vi "laserChangePara.vi"(7 "LaserProp":T1, 8 "error in (no error)":errorcluster, 9 "LaserMode":string, 10 "LaserON":bool, 11 "LaserPow":dbl) -> (0 "error out":errorcluster, 2 "String":string, 3 "Boolean":bool)   [LabVIEW 2021]
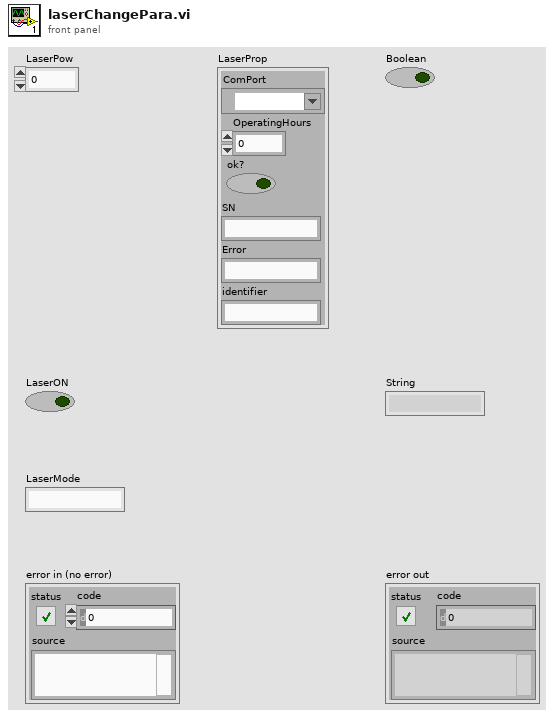
[diagram p1: front panel]
types:
  T1 = cluster{"ComPort":refnum<visa-resource-name>, "OperatingHours":dbl, "ok?":bool, "SN":string, "Error":string, "identifier":string}
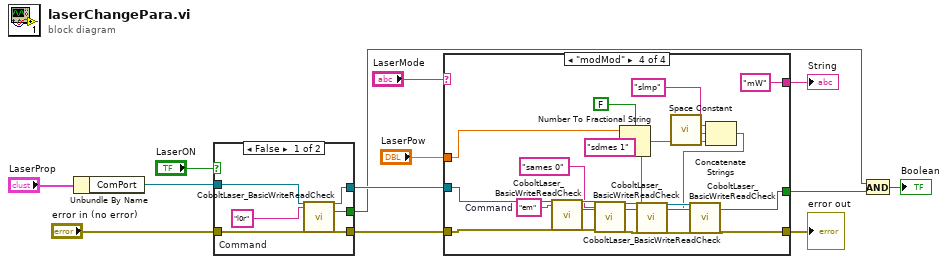
[diagram p0: block diagram]
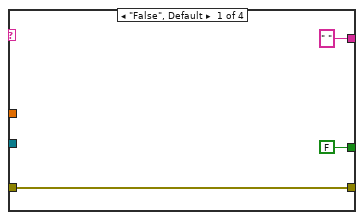
[diagram p2: hidden frame]
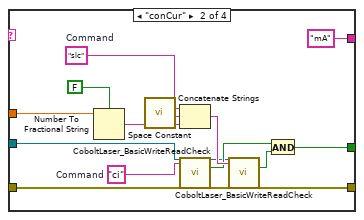
[diagram p3: hidden frame]
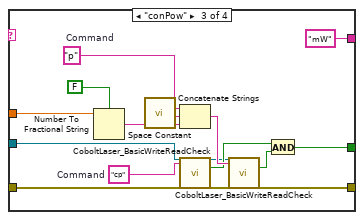
[diagram p4: hidden frame]
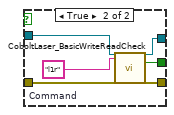
[diagram p5: hidden frame]
diagram:
  n1 = Unbundle By Name("LaserProp") -> ("ComPort"=w3:refnum<visa-resource-name>)
  n2 = case shown="False" "LaserON" {
    tunnel: "error in (no error)" -> [w17 w23]
    tunnel: w3 -> [w18 w24]
    tunnel: [w15 w22] -> w10
    tunnel: [w14 w21] -> w11
    tunnel: [w16 w20] -> w12
    frame False {
      w19 = "l0r"  # Command
      n3 = call "CoboltLaser_BasicWriteReadCheck.vi"("ComPort"=w18, "Command"=w19, "error in (no error)"=w17) -> ("ComPortOut"=w14:refnum<visa-resource-name>, "ResponseOK"=w15:bool, "error out"=w16:errorcluster)  [unwired: 21 in, 1 out]
    }
    frame True {
      w25 = "l1r"  # Command
      n4 = call "CoboltLaser_BasicWriteReadCheck.vi"("ComPort"=w24, "Command"=w25, "error in (no error)"=w23) -> ("ComPortOut"=w21:refnum<visa-resource-name>, "ResponseOK"=w22:bool, "error out"=w20:errorcluster)  [unwired: 21 in, 1 out]
    }
  }
  n5 = case shown="\"modMod\"" "LaserMode" {
    tunnel: w12 -> [w27 w33 w60 w77]
    tunnel: "LaserPow" -> [_ w30 w54 w63]
    tunnel: [FALSE w29 w49 w76] -> w8
    tunnel: [w27 w32 w48 w69] -> w7
    tunnel: w11 -> [_ w31 w47 w78]
    tunnel: [" " "mA" "mW" "mW"] -> w13
    frame "False", Default {
    }
    frame "conCur" {
      w42 = "slc"  # Command
      w43 = "ci"  # Command
      n6 = Number To Fractional String(use system decimal point (T)=FALSE, number=w30) -> (F-format string=w39:string)  [unwired: 2 in]
      n7 = call <vilib>:"Space Constant.vi"() -> ("String"=w40:string)
      n8 = Concatenate Strings(w42, w40, w39) -> (w38:string)
      n9 = call "CoboltLaser_BasicWriteReadCheck.vi"("ComPort"=w31, "Command"=w43, "error in (no error)"=w33) -> ("ComPortOut"=w34:refnum<visa-resource-name>, "ResponseOK"=w35:bool, "error out"=w37:errorcluster)  [unwired: 21 in, 1 out]
      n10 = call "CoboltLaser_BasicWriteReadCheck.vi"("ComPort"=w34, "Command"=w38, "error in (no error)"=w37) -> ("ResponseOK"=w36:bool, "error out"=w32:errorcluster)  [unwired: 21 in, 2 out]
      n11 = And(x=w35, y=w36) -> (x .and. y?=w29:bool)
    }
    frame "conPow" {
      w58 = "p"  # Command
      w59 = "cp"  # Command
      n12 = Number To Fractional String(use system decimal point (T)=FALSE, number=w54) -> (F-format string=w55:string)  [unwired: 2 in]
      n13 = call <vilib>:"Space Constant.vi"() -> ("String"=w56:string)
      n14 = Concatenate Strings(w58, w56, w55) -> (w53:string)
      n15 = call "CoboltLaser_BasicWriteReadCheck.vi"("ComPort"=w47, "Command"=w59, "error in (no error)"=w60) -> ("ComPortOut"=w46:refnum<visa-resource-name>, "ResponseOK"=w50:bool, "error out"=w52:errorcluster)  [unwired: 21 in, 1 out]
      n16 = call "CoboltLaser_BasicWriteReadCheck.vi"("ComPort"=w46, "Command"=w53, "error in (no error)"=w52) -> ("ResponseOK"=w51:bool, "error out"=w48:errorcluster)  [unwired: 21 in, 2 out]
      n17 = And(x=w50, y=w51) -> (x .and. y?=w49:bool)
    }
    frame "modMod" {
      w79 = "em"  # Command
      n18 = call "CoboltLaser_BasicWriteReadCheck.vi"("ComPort"=w78, "Command"=w79, "error in (no error)"=w77) -> ("ComPortOut"=w75:refnum<visa-resource-name>, "ResponseOK"=w76:bool, "error out"=w74:errorcluster)  [unwired: 21 in, 1 out]
      n19 = call "CoboltLaser_BasicWriteReadCheck.vi"("ComPort"=w75, "Command"="sames 0", "error in (no error)"=w74) -> ("ComPortOut"=w72:refnum<visa-resource-name>, "error out"=w71:errorcluster)  [unwired: 21 in, 2 out]
      n20 = Number To Fractional String(use system decimal point (T)=FALSE, number=w63) -> (F-format string=w64:string)  [unwired: 2 in]
      n21 = call "CoboltLaser_BasicWriteReadCheck.vi"("ComPort"=w72, "Command"="sdmes 1", "error in (no error)"=w71) -> ("ComPortOut"=w67:refnum<visa-resource-name>, "error out"=w68:errorcluster)  [unwired: 21 in, 2 out]
      n22 = call <vilib>:"Space Constant.vi"() -> ("String"=w65:string)
      n23 = Concatenate Strings("slmp" ("string"), w65, w64) -> (w62:string)
      n24 = call "CoboltLaser_BasicWriteReadCheck.vi"("ComPort"=w67, "Command"=w62, "error in (no error)"=w68) -> ("error out"=w69:errorcluster)  [unwired: 21 in, 3 out]
    }
  }
  "String" <- w13
  "error out" <- w7
  n25 = And(x=w10, y=w8) -> (x .and. y?=→"Boolean":bool)
